vi "JYMoveToWavelength.vi"(3 "error in (no error)":errorcluster, 4 "Target WL":dbl, 5 "UniqueID":string, 6 "RefNum In":refnum<k7>) -> (0 "error out":errorcluster, 1 "IsBusy":bool, 2 "Refnum Out":refnum<k7>)   [LabVIEW 2009]
doc: "JYMoveToWavelength.vi\n\nMoves the mono to a new wavelength.\n\nInputs\nMono RefNum - the LabView automation refnum of the mono\nTarget Wavelength - double; new wavelength for mono\nError Cluster\n\n\nOutputs\nError Cluster"
panel:
  out "UseUniqueID":bool
  in  "Mode Select":bool
  # "Local / Front Panel Mode"
  # "Remote / Progam Mode"
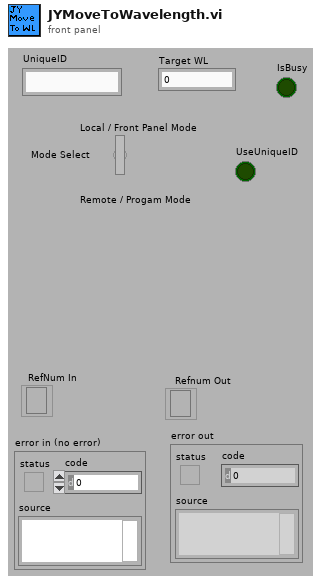
[diagram p1: front panel]
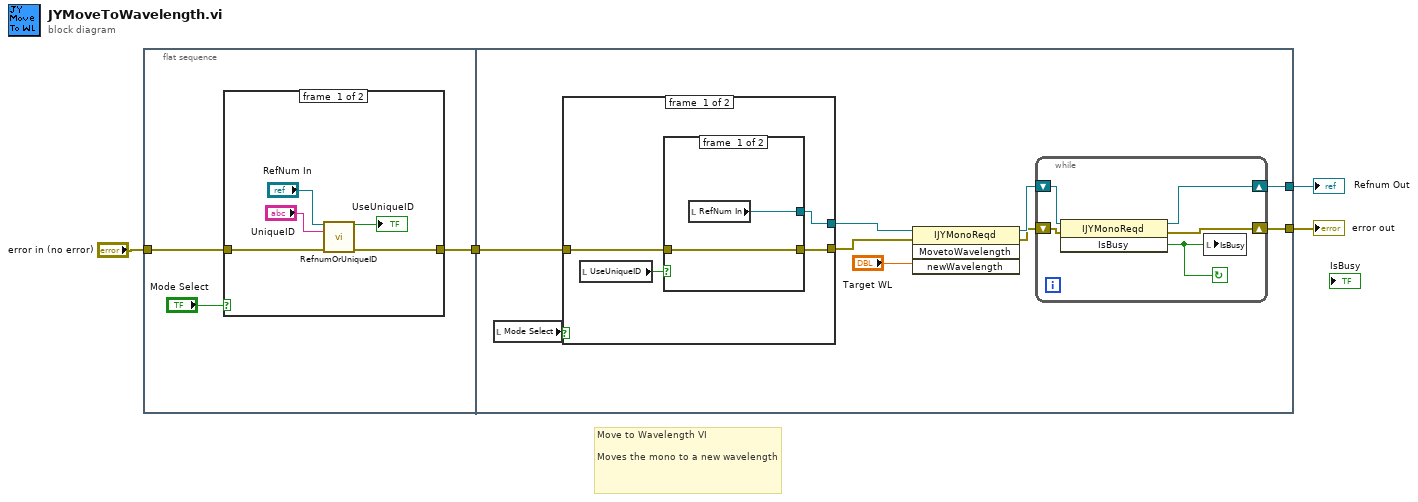
[diagram p0: block diagram]
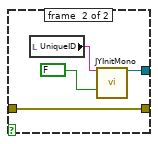
[diagram p3: hidden frame]
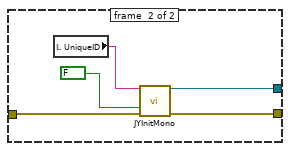
[diagram p4: hidden frame]
diagram:
  # "Move to Wavelength VI\n\nMoves the mono to a new wavelength"
  n1 = flat-sequence {
    tunnel: "error in (no error)" -> [w6]
    tunnel: [w5] -> w3
    tunnel: w3 -> [w19]
    tunnel: [w16] -> w2
    tunnel: [w15] -> w1
    frame #0 {
      n2 = case shown="False" "Mode Select" {
        tunnel: w6 -> [w9 w13]
        tunnel: [w8 w13] -> w5
        frame #0 {
          n3 = call "RefnumOrUniqueID.vi"("Refnum IN"="RefNum In", "String in"="UniqueID", "error in (no error)"=w9) -> ("UseUniqueID"=→"UseUniqueID":bool, "error out"=w8:errorcluster)  [unwired: 11 out]
        }
        frame #1 {
        }
      }
    }
    frame #1 {
      n4 = local read "Mode Select"() -> (w22:bool)
      n5 = case shown="False" w22 {
        tunnel: [w30 w40] -> w20
        tunnel: w19 -> [w29 w39]
        tunnel: [w28 w38] -> w18
        frame #0 {
          n6 = local read "UseUniqueID"() -> (w31:bool)
          n7 = case shown="False" w31 {
            tunnel: [w33 w35] -> w30
            tunnel: w29 -> [w32 w34]
            tunnel: [w32 w34] -> w28
            frame #0 {
              n8 = local read "RefNum In"() -> (w33:refnum<k7>)
            }
            frame #1 {
              n9 = local read "UniqueID"() -> (w37:string)
              n10 = call "JYInitMono.vi"("Unique ID"=w37, "Force Init"=FALSE) -> ("Mono RefNum out"=w35:refnum<k7>)  [unwired: 2 in, 11 out]
            }
          }
        }
        frame #1 {
          n11 = local read "UniqueID"() -> (w42:string)
          n12 = call "JYInitMono.vi"("Unique ID"=w42, "Force Init"=FALSE, "error in (no error)"=w39) -> ("Mono RefNum out"=w40:refnum<k7>, "error out"=w38:errorcluster)  [unwired: 1 in, 10 out]
        }
      }
      n13 = invoke class="IJYMonoReqd" method="MovetoWavelength"(reference=w20, error in=w18, "newWavelength"="Target WL") -> (reference out=w21:refnum<k7>, error out=w17:errorcluster)  [unwired: 1 in, 2 out]
      n14 = while {
        shift-right: [w23] -> w15
        shift-left: w17 -> [w25]
        shift-right: [w24] -> w16
        shift-left: w21 -> [w26]
        stop <- w27 continue-if-true
        n15 = invoke class="IJYMonoReqd" method="IsBusy"(reference=w26, error in=w25) -> (reference out=w24:refnum<k7>, error out=w23:errorcluster, "IsBusy"=w27:bool)  [unwired: 1 in]
        n16 = local write "IsBusy"(w27) -> ()
      }
    }
  }
  "error out" <- w1
  "Refnum Out" <- w2
